vi "NIDAQControl2.vi"() -> ()   [LabVIEW 2015]
uses:
  <vilib>/DAQmx/write.llb/DAQmx Write (Analog 1D Wfm NChan NSamp).vi
  <vilib>/DAQmx/miscellaneous.llb/DAQmx Fill In Error Info.vi
panel:
  out "time":dbl
  out "Numeric":i32
  in  "stop":bool
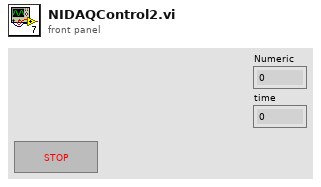
[diagram p1: front panel]
types:
  T1 = typedef "Rendezvous RefNum" = refnum<k1>
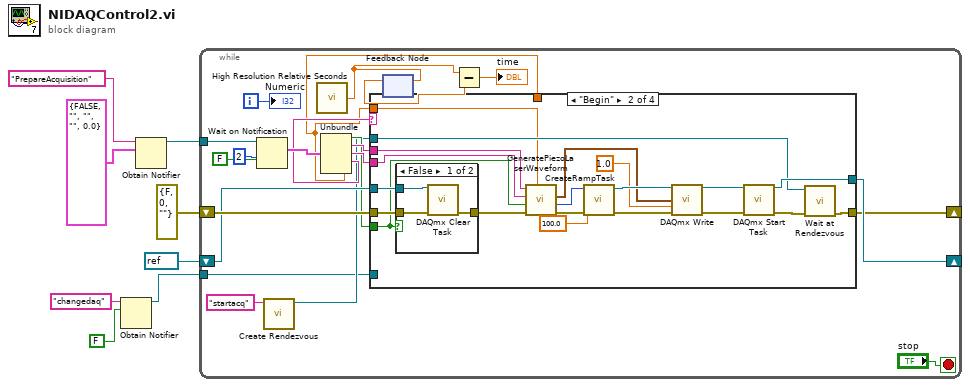
[diagram p0: block diagram]
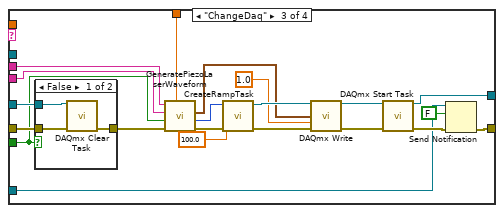
[diagram p4: hidden frame]
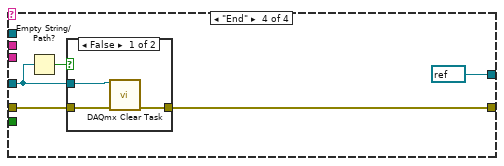
[diagram p6: hidden frame]
diagram:
  n1 = Obtain Notifier(name (unnamed)="changedaq", notification data type=FALSE) -> (notifier out=w1:refnum<notifier>)  [unwired: 2 in, 2 out]
  n2 = Obtain Notifier(name (unnamed)="PrepareAcquisition", notification data type=cluster{bool, string, string, string, dbl} {FALSE, "", "", "", 0.0}) -> (notifier out=w6:refnum<notifier>)  [unwired: 2 in, 2 out]
  n3 = while {
    tunnel: w6 -> [w28]
    shift-right: [w22] -> _
    shift-left: refnum<k21> refnum ("task out") -> [w19]
    shift-right: [w21] -> _
    shift-left: errorcluster {"status"=FALSE, "code"=0, "source"=""} ("error out") -> [w24]
    tunnel: w1 -> [w13]
    i -> [w18]
    stop <- "stop" stop-if-true
    n4 = Wait on Notification(notifier=w28, ignore previous (F)=FALSE, timeout in ms (-1)=2) -> (notification=w29:cluster{bool, string, string, string, dbl})  [unwired: 1 in, 3 out]
    n5 = call <vilib>:"Create Rendezvous.vi"("name (unnamed)"="startacq") -> ("rendezvous"=w15:T1)  [unwired: 4 in, 2 out]
    n6 = call <vilib>:"High Resolution Relative Seconds.vi"() -> ("relative seconds"=w12:dbl)
    n7 = Unbundle(w29) -> (w17:bool, w26:string, w25:string, w23:string, w9:dbl)
    n8 = case shown="\"Begin\"" w23 {
      tunnel: w26 -> [_ w51 w76 _]
      tunnel: w25 -> [_ w50 w75 _]
      tunnel: w17 -> [_ w37 w62 _]
      tunnel: w24 -> [w30 w44 w69 w85]
      tunnel: [w31 w38 w63 refnum<k21> refnum ("task out")] -> w22
      tunnel: [w30 w35 w60 w84] -> w21
      tunnel: w19 -> [w31 w45 w70 w82]
      tunnel: w15 -> [_ w34 _ _]
      tunnel: w13 -> [_ _ w59 _]
      tunnel: w9 -> [_ w33 _ _]
      tunnel: w9 -> [_ _ w57 _]
      frame "Continue", Default {
      }
      frame "Begin" {
        n9 = case shown="False" w37 {
          tunnel: w45 -> [w54 _]
          tunnel: w44 -> [w53 w55]
          tunnel: [w52 w55] -> w43
          frame False {
            n10 = call <vilib>:"DAQmx Clear Task.vi"("task in"=w54, "error in"=w53) -> ("error out"=w52:errorcluster)  [unwired: 13 in]
          }
          frame True {
          }
        }
        n11 = call "GeneratePiezoLaserWaveform.vi"("Acquition Time (sec)"=w33, "error out"=w43, "Start or Continue?"=w37, "Piezo Mode"=w50, "Laser Mode"=w51) -> ("error out"=w48:errorcluster, "Number of Samples"=w49:i32, "Waveforms"=w41:waveform(dbl)[])  [unwired: 4 in]
        n12 = call "CreateRampTask.vi"("error in"=w48, "Sample Rate"=100.0, "Number of Samples"=w49) -> ("error out"=w47:errorcluster, "task out"=w46:refnum<k21>)  [unwired: 7 in]
        n13 = call-poly <vilib>:"DAQmx Write.vi"("task/channels in"=w46, "data"=w41, "timeout"=1.0, "error in"=w47) -> ("task out"=w39:refnum<k21>, "error out"=w42:errorcluster)  [unwired: 9 in, 1 out]
        n14 = call <vilib>:"DAQmx Start Task.vi"("task/channels in"=w39, "error in"=w42) -> ("task out"=w38:refnum<k21>, "error out"=w36:errorcluster)  [unwired: 12 in]
        n15 = call <vilib>:"Wait at Rendezvous.vi"("error in (no error)"=w36, "rendezvous"=w34) -> ("error out"=w35:errorcluster)  [unwired: 3 in, 2 out]
      }
      frame "ChangeDaq" {
        n16 = case shown="False" w62 {
          tunnel: w70 -> [w79 _]
          tunnel: w69 -> [w78 w80]
          tunnel: [w77 w80] -> w68
          frame False {
            n17 = call <vilib>:"DAQmx Clear Task.vi"("task in"=w79, "error in"=w78) -> ("error out"=w77:errorcluster)  [unwired: 13 in]
          }
          frame True {
          }
        }
        n18 = call "GeneratePiezoLaserWaveform.vi"("Acquition Time (sec)"=w57, "error out"=w68, "Start or Continue?"=w62, "Piezo Mode"=w75, "Laser Mode"=w76) -> ("error out"=w73:errorcluster, "Number of Samples"=w74:i32, "Waveforms"=w66:waveform(dbl)[])  [unwired: 4 in]
        n19 = call "CreateRampTask.vi"("error in"=w73, "Sample Rate"=100.0, "Number of Samples"=w74) -> ("error out"=w72:errorcluster, "task out"=w71:refnum<k21>)  [unwired: 7 in]
        n20 = call-poly <vilib>:"DAQmx Write.vi"("task/channels in"=w71, "data"=w66, "timeout"=1.0, "error in"=w72) -> ("task out"=w64:refnum<k21>, "error out"=w67:errorcluster)  [unwired: 9 in, 1 out]
        n21 = call <vilib>:"DAQmx Start Task.vi"("task/channels in"=w64, "error in"=w67) -> ("task out"=w63:refnum<k21>, "error out"=w61:errorcluster)  [unwired: 12 in]
        n22 = Send Notification(notification=FALSE, notifier=w59, error in (no error)=w61) -> (error out=w60:errorcluster)  [unwired: 1 out]
      }
      frame "End" {
        n23 = Empty String/Path?(string/path=w82) -> (empty?=w81:bool)
        n24 = case shown="False" w81 {
          tunnel: w85 -> [w88 w89]
          tunnel: [w87 w89] -> w84
          tunnel: w82 -> [w86 _]
          frame False {
            n25 = call <vilib>:"DAQmx Clear Task.vi"("task in"=w86, "error in"=w88) -> ("error out"=w87:errorcluster)  [unwired: 13 in]
          }
          frame True {
          }
        }
      }
    }
    n26 = feedback-in #1(w12) -> ()
    n27 = feedback #1() -> (w11:dbl)  [unwired: 1 in]
    n28 = Subtract(x=w12, y=w11) -> (x-y=→"time":dbl)
    "Numeric" <- w18
  }
